vi "LRU Check.vi"(11 "State in":cluster{"Hallway":string[], "Rooms":string[][]}) -> (2 "LRU Check Result":cluster{"Key Not Found?":bool, "Value":u64}, 3 "State out":cluster{"Hallway":string[], "Rooms":string[][]})   [LabVIEW 2019, in "23.lvlib"]
uses:
  23.lvlib
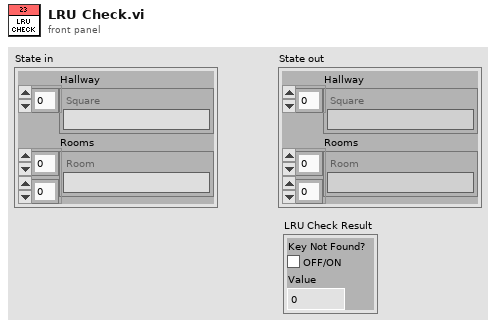
[diagram p1: front panel]
types:
  T1 = cluster{"Stop":bool, "Check":bool, "Key":cluster{"Hallway":string[], "Rooms":string[][]}, "Value":u64, "Check Notifier":refnum<notifier>}
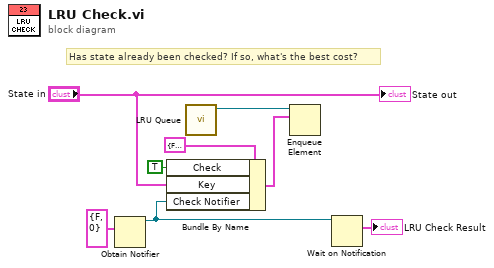
[diagram p0: block diagram]
diagram:
  # "Has state already been checked? If so, what's the best cost?"
  n1 = Obtain Notifier(notification data type=cluster{"Key Not Found?":bool, "Value":u64} {"Key Not Found?"=FALSE, "Value"=0}) -> (notifier out=w8:refnum<notifier>)  [unwired: 3 in, 2 out]
  n2 = Bundle By Name(cluster=T1 {"Stop"=FALSE, "Check"=FALSE, "Key"={"Hallway"=[], "Rooms"=[]}, "Value"=0, "Check Notifier"=refnum}, "Check"=TRUE, "Key"="State in", "Check Notifier"=w8) -> (w5:T1)
  n3 = call "LRU Queue.vi"() -> ("LRU Queue"=w4:refnum<queue>)  [unwired: 11 in]
  n4 = Enqueue Element(queue=w4, element=w5) -> ()  [unwired: 2 in, 3 out]
  n5 = Wait on Notification(notifier=w8) -> (notification=→"LRU Check Result":cluster{"Key Not Found?":bool, "Value":u64})  [unwired: 3 in, 3 out]
  "State out" <- "State in"
